vi "Read Setpoint.vi"(8 "error in (no error)":errorcluster, 11 "Lakeshore 336 in":refnum<class "Lakeshore 336.lvclass">) -> (0 "error out":errorcluster, 2 "Setpoint":dbl[](array[numeric]), 3 "Lakeshore 336 out":refnum<class "Lakeshore 336.lvclass">)   [LabVIEW 2022 SP3, in "Lakeshore 336.lvclass"]
uses:
  Lakeshore 336.lvclass
  Temp Control.lvclass
  Lakeshore 336.lvclass/Lakeshore 336.ctl
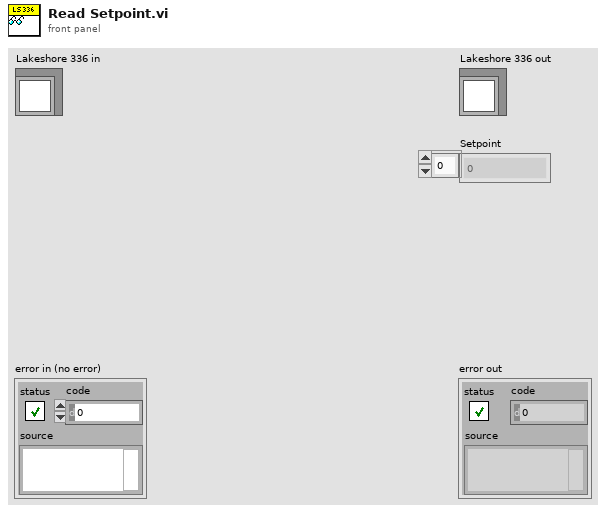
[diagram p1: front panel]
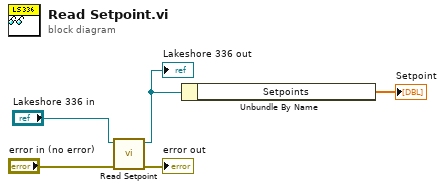
[diagram p0: block diagram]
diagram:
  n1 = call-parent "Read Setpoint.vi"("error in (no error)"="error in (no error)", "Temp Control in"="Lakeshore 336 in") -> ("error out"=→"error out":errorcluster, "Temp Control out"=w2:refnum<class "Lakeshore 336.lvclass">)  [unwired: 7 in, 1 out]
  "Lakeshore 336 out" <- w2
  n2 = Unbundle By Name(w2) -> ("Setpoints"=→"Setpoint":dbl[])
